vi "CAL TimeOut.vi"(5 "CAL-Start":timestamp, 7 "im Bereich seit":timestamp, 10 "im Bereich":bool) -> (0 "im Bereich seit (Ausgang)":timestamp, 2 "Sekunden seit CAL-Start":sgl, 3 "Sekunden im Bereich":sgl)   [LabVIEW 2020, in "ABB-EL3000.lvlib" / "Allgemeine VI.lvlib"]
uses:
  Allgemeine VI.lvlib
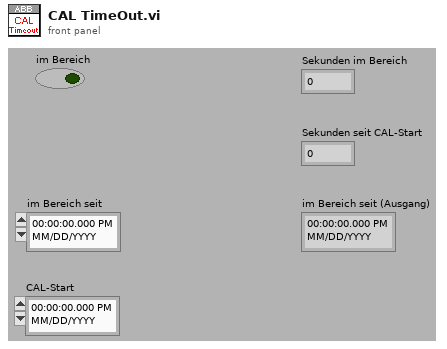
[diagram p1: front panel]
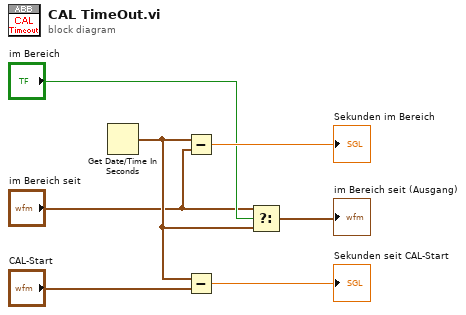
[diagram p0: block diagram]
diagram:
  n1 = Get Date/Time In Seconds() -> (seconds since 1Jan1904=w3:timestamp)
  n2 = Subtract(x=w3, y="im Bereich seit") -> (x-y=→"Sekunden im Bereich":dbl)
  n3 = Subtract(x=w3, y="CAL-Start") -> (x-y=→"Sekunden seit CAL-Start":dbl)
  n4 = Select(t="im Bereich seit", s="im Bereich", f=w3) -> (s? t:f=→"im Bereich seit (Ausgang)":timestamp)
